vi "Register with Dispatcher.vi"(8 "error in (no error)":errorcluster, 11 "Worker in":refnum<class "Worker.lvclass">) -> (0 "error out":errorcluster, 3 "Worker out":refnum<class "Worker.lvclass">)   [LabVIEW 2023, in "Worker.lvlib" / "Worker.lvclass"]
doc: "Notify the Incoming Work Dispatcher that this Worker is available to be assigned a task."
uses:
  Worker.lvclass
  c:/dev/_r/4/eng/lv-core/lvpostprocessingd/lv_mc_x86_64/dist_i386/vi.lib/ActorFramework/Actor/Actor.lvclass
  <vilib>/ActorFramework/Actor/Actor.lvclass/Actor.ctl
  <vilib>/ActorFramework/Message Enqueuer/Message Enqueuer.lvclass/Message Enqueuer.ctl
  Worker.lvclass/Worker.ctl
  Work Dispatcher Messages/Add Available Worker Msg/Add Available Worker Msg.lvclass/Add Available Worker Msg.ctl
  <vilib>/ActorFramework/Message Enqueuer/Init from Existing Queue.vi
  <vilib>/ActorFramework/Message Enqueuer/Enqueue.vi
  Work Dispatcher Messages/Add Available Worker Msg/Add Available Worker Msg.lvclass
  c:/dev/_r/4/eng/lv-core/lvpostprocessingd/lv_mc_x86_64/dist_i386/vi.lib/ActorFramework/Message/Message.lvclass
  <vilib>/ActorFramework/Message Priority Queue/Priority Enqueue.vi
  <vilib>/ActorFramework/Message Enqueuer/Message Enqueuer.lvclass
  <vilib>/ActorFramework/Actor/Actor.lvclass
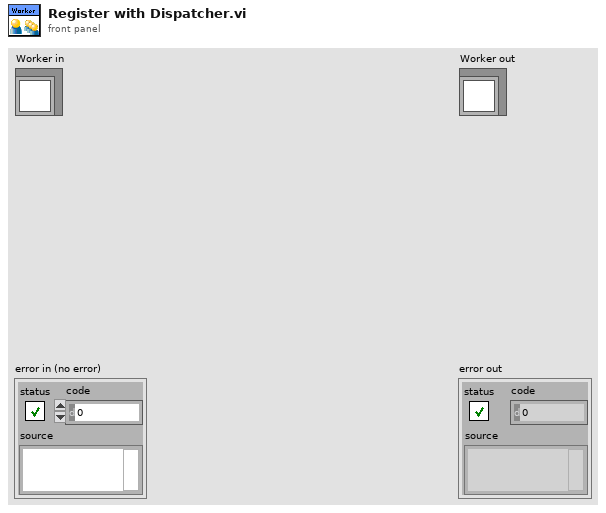
[diagram p1: front panel]
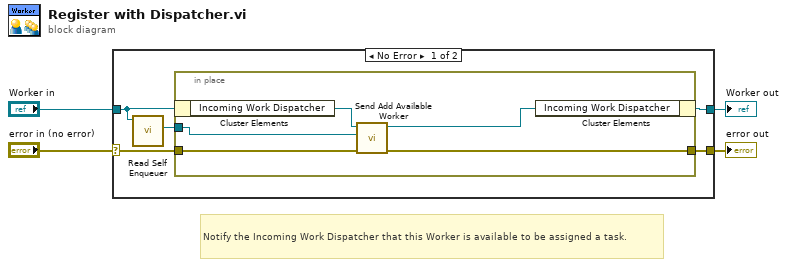
[diagram p0: block diagram]
diagram:
  # "Notify the Incoming Work Dispatcher that this Worker is available to be assigned a task."
  n1 = case shown="No Error" "error in (no error)" {
    selector: "error in (no error)" -> [w7 w16]
    tunnel: [w6 w16] -> w3
    tunnel: [w5 w15] -> w1
    tunnel: "Worker in" -> [w9 w15]
    frame No Error {
      n2 = call <vilib>:"Read Self Enqueuer.vi"("Actor"=w9) -> ("Self Enqueuer"=w8:refnum<class "Message Enqueuer.lvclass">)  [unwired: 10 in]
      n3 = in-place "In Place Element Structure" {
        in-place-border: w8 -> [w12]
        in-place-border: w7 -> [w11]
        in-place-border: [w10] -> w6
        n4 = in-place-cluster #1 ("Unbundle / Bundle Elements")(w9) -> ("Incoming Work Dispatcher"=w14:refnum<class "Message Enqueuer.lvclass">)
        n5 = call "Send Add Available Worker.vi"("error in (no error)"=w11, "Worker"=w12, "Message Enqueuer"=w14) -> ("error out"=w10:errorcluster, "Message Enqueuer out"=w13:refnum<class "Message Enqueuer.lvclass">)  [unwired: 7 in]
        n6 = in-place-cluster #1 ("Unbundle / Bundle Elements")("Incoming Work Dispatcher"=w13) -> (w5:refnum<class "Worker.lvclass">)
      }
    }
    frame Error {
    }
  }
  "error out" <- w3
  "Worker out" <- w1
